vi "S4GUI.vi"(7 "Tab ObsEng":enum32{"Obs", "CCD modes", "Guider", "Eng"}(tab)) -> ()   [LabVIEW 2018] (continued)
            n1734 = call-dynamic "Read State Machine.vi"("error in (no error)"=w3186, "Device in"=w3187) -> ("error out"=w3286:errorcluster, "State Machine.lvclass"=w3288:refnum<class "State Machine.lvclass">, "Device out"=w3289:refnum<class "Channel.lvclass">)  [unwired: 7 in]
            n1735 = call-dynamic "Write State.vi"("error in (no error)"=w3286, "State"=60, "State Machine in"=w3288) -> ("error out"=w3285:errorcluster, "State Machine out"=w3287:refnum<class "State Machine.lvclass">)  [unwired: 7 in]
            n1736 = call-dynamic "Write State Machine.vi"("error in (no error)"=w3285, "State Machine.lvclass"=w3287, "Device in"=w3289) -> ("error out"=w3282:errorcluster, "Device out"=w3283:refnum<class "Channel.lvclass">)  [unwired: 7 in]
            n1737 = call-dynamic "Write Channel.vi"("error in (no error)"=w3282, "Channel.lvclass"=w3283, "Acquisition in"=w3291) -> ("error out"=w3281:errorcluster, "Acquisition out"=w3280:refnum<class "Acquisition.lvclass">)  [unwired: 7 in]
            n1738 = call-dynamic "Write AcquisitionA.vi"("error in (no error)"=w3281, "Acquisition.lvclass"=w3280, "S4ACS_GUI in"=w3293) -> ("error out"=w3217:errorcluster, "S4ACS_GUI out"=w3216:refnum<class "S4GUI.lvclass">)  [unwired: 7 in]
            n1739 = call "Read AcquisitionB.vi"("error in (no error)"=w3217, "S4ACS_GUI in"=w3216) -> ("error out"=w3259:errorcluster, "Acquisition.lvclass"=w3257:refnum<class "Acquisition.lvclass">, "S4ACS_GUI out"=w3256:refnum<class "S4GUI.lvclass">)  [unwired: 7 in]
            n1740 = call-dynamic "Read Channel.vi"("error in (no error)"=w3259, "Acquisition in"=w3257) -> ("error out"=w3272:errorcluster, "Channel.lvclass"=w3270:refnum<class "Channel.lvclass">, "Acquisition out"=w3258:refnum<class "Acquisition.lvclass">)  [unwired: 7 in]
            n1741 = call "Write section_name.vi"("error in (no error)"=w3272, "section_name"="CCD_ACS2", "Channel in"=w3270) -> ("error out"=w3273:errorcluster, "Channel out"=w3271:refnum<class "Channel.lvclass">)  [unwired: 7 in]
            n1742 = call-dynamic "load config.vi"("error in (no error)"=w3273, "cfg file name"=w3206, "Channel in"=w3271) -> ("error out"=w3201:errorcluster, "Channel out"=w3199:refnum<class "Channel.lvclass">)  [unwired: 7 in]
            n1743 = call-dynamic "save config.vi"("error in (no error)"=w3201, "file config"="lastsaved.cfg", "Channel in"=w3199) -> ("error out"=w3200:errorcluster, "Channel out"=w3198:refnum<class "Channel.lvclass">)  [unwired: 7 in]
            n1744 = call-dynamic "Read State Machine.vi"("error in (no error)"=w3200, "Device in"=w3198) -> ("error out"=w3263:errorcluster, "State Machine.lvclass"=w3261:refnum<class "State Machine.lvclass">, "Device out"=w3260:refnum<class "Channel.lvclass">)  [unwired: 7 in]
            n1745 = call-dynamic "Write State.vi"("error in (no error)"=w3263, "State"=60, "State Machine in"=w3261) -> ("error out"=w3264:errorcluster, "State Machine out"=w3262:refnum<class "State Machine.lvclass">)  [unwired: 7 in]
            n1746 = call-dynamic "Write State Machine.vi"("error in (no error)"=w3264, "State Machine.lvclass"=w3262, "Device in"=w3260) -> ("error out"=w3267:errorcluster, "Device out"=w3266:refnum<class "Channel.lvclass">)  [unwired: 7 in]
            n1747 = call-dynamic "Write Channel.vi"("error in (no error)"=w3267, "Channel.lvclass"=w3266, "Acquisition in"=w3258) -> ("error out"=w3268:errorcluster, "Acquisition out"=w3269:refnum<class "Acquisition.lvclass">)  [unwired: 7 in]
            n1748 = call "Write AcquisitionB.vi"("error in (no error)"=w3268, "Acquisition.lvclass"=w3269, "S4ACS_GUI in"=w3256) -> ("error out"=w3215:errorcluster, "S4ACS_GUI out"=w3214:refnum<class "S4GUI.lvclass">)  [unwired: 7 in]
            n1749 = call-dynamic "Read AcquisitionC.vi"("error in (no error)"=w3215, "S4ACS_GUI in"=w3214) -> ("error out"=w3252:errorcluster, "Acquisition.lvclass"=w3254:refnum<class "Acquisition.lvclass">, "S4ACS_GUI out"=w3255:refnum<class "S4GUI.lvclass">)  [unwired: 7 in]
            n1750 = call-dynamic "Read Channel.vi"("error in (no error)"=w3252, "Acquisition in"=w3254) -> ("error out"=w3239:errorcluster, "Channel.lvclass"=w3241:refnum<class "Channel.lvclass">, "Acquisition out"=w3253:refnum<class "Acquisition.lvclass">)  [unwired: 7 in]
            n1751 = call "Write section_name.vi"("error in (no error)"=w3239, "section_name"="CCD_ACS3", "Channel in"=w3241) -> ("error out"=w3238:errorcluster, "Channel out"=w3240:refnum<class "Channel.lvclass">)  [unwired: 7 in]
            n1752 = call-dynamic "load config.vi"("error in (no error)"=w3238, "cfg file name"=w3206, "Channel in"=w3240) -> ("error out"=w3196:errorcluster, "Channel out"=w3194:refnum<class "Channel.lvclass">)  [unwired: 7 in]
            n1753 = call-dynamic "save config.vi"("error in (no error)"=w3196, "file config"="lastsaved.cfg", "Channel in"=w3194) -> ("error out"=w3195:errorcluster, "Channel out"=w3193:refnum<class "Channel.lvclass">)  [unwired: 7 in]
            n1754 = call-dynamic "Read State Machine.vi"("error in (no error)"=w3195, "Device in"=w3193) -> ("error out"=w3248:errorcluster, "State Machine.lvclass"=w3250:refnum<class "State Machine.lvclass">, "Device out"=w3251:refnum<class "Channel.lvclass">)  [unwired: 7 in]
            n1755 = call-dynamic "Write State.vi"("error in (no error)"=w3248, "State"=60, "State Machine in"=w3250) -> ("error out"=w3247:errorcluster, "State Machine out"=w3249:refnum<class "State Machine.lvclass">)  [unwired: 7 in]
            n1756 = call-dynamic "Write State Machine.vi"("error in (no error)"=w3247, "State Machine.lvclass"=w3249, "Device in"=w3251) -> ("error out"=w3244:errorcluster, "Device out"=w3245:refnum<class "Channel.lvclass">)  [unwired: 7 in]
            n1757 = call-dynamic "Write Channel.vi"("error in (no error)"=w3244, "Channel.lvclass"=w3245, "Acquisition in"=w3253) -> ("error out"=w3243:errorcluster, "Acquisition out"=w3242:refnum<class "Acquisition.lvclass">)  [unwired: 7 in]
            n1758 = call-dynamic "Write AcquisitionC.vi"("error in (no error)"=w3243, "Acquisition.lvclass"=w3242, "S4ACS_GUI in"=w3255) -> ("error out"=w3213:errorcluster, "S4ACS_GUI out"=w3212:refnum<class "S4GUI.lvclass">)  [unwired: 7 in]
            n1759 = call-dynamic "Read AcquisitionD.vi"("error in (no error)"=w3213, "S4ACS_GUI in"=w3212) -> ("error out"=w3221:errorcluster, "Acquisition.lvclass"=w3219:refnum<class "Acquisition.lvclass">, "S4ACS_GUI out"=w3218:refnum<class "S4GUI.lvclass">)  [unwired: 7 in]
            n1760 = call-dynamic "Read Channel.vi"("error in (no error)"=w3221, "Acquisition in"=w3219) -> ("error out"=w3234:errorcluster, "Channel.lvclass"=w3232:refnum<class "Channel.lvclass">, "Acquisition out"=w3220:refnum<class "Acquisition.lvclass">)  [unwired: 7 in]
            n1761 = call "Write section_name.vi"("error in (no error)"=w3234, "section_name"="CCD_ACS4", "Channel in"=w3232) -> ("error out"=w3235:errorcluster, "Channel out"=w3233:refnum<class "Channel.lvclass">)  [unwired: 7 in]
            n1762 = call-dynamic "load config.vi"("error in (no error)"=w3235, "cfg file name"=w3206, "Channel in"=w3233) -> ("error out"=w3192:errorcluster, "Channel out"=w3190:refnum<class "Channel.lvclass">)  [unwired: 7 in]
            n1763 = call-dynamic "save config.vi"("error in (no error)"=w3192, "file config"="lastsaved.cfg", "Channel in"=w3190) -> ("error out"=w3191:errorcluster, "Channel out"=w3189:refnum<class "Channel.lvclass">)  [unwired: 7 in]
            n1764 = call-dynamic "Read State Machine.vi"("error in (no error)"=w3191, "Device in"=w3189) -> ("error out"=w3225:errorcluster, "State Machine.lvclass"=w3223:refnum<class "State Machine.lvclass">, "Device out"=w3222:refnum<class "Channel.lvclass">)  [unwired: 7 in]
            n1765 = call-dynamic "Write State.vi"("error in (no error)"=w3225, "State"=60, "State Machine in"=w3223) -> ("error out"=w3226:errorcluster, "State Machine out"=w3224:refnum<class "State Machine.lvclass">)  [unwired: 7 in]
            n1766 = call-dynamic "Write State Machine.vi"("error in (no error)"=w3226, "State Machine.lvclass"=w3224, "Device in"=w3222) -> ("error out"=w3229:errorcluster, "Device out"=w3228:refnum<class "Channel.lvclass">)  [unwired: 7 in]
            n1767 = call-dynamic "Write Channel.vi"("error in (no error)"=w3229, "Channel.lvclass"=w3228, "Acquisition in"=w3220) -> ("error out"=w3230:errorcluster, "Acquisition out"=w3231:refnum<class "Acquisition.lvclass">)  [unwired: 7 in]
            n1768 = call-dynamic "Write AcquisitionD.vi"("error in (no error)"=w3230, "Acquisition.lvclass"=w3231, "S4ACS_GUI in"=w3218) -> ("error out"=w3209:errorcluster, "S4ACS_GUI out"=w3211:refnum<class "S4GUI.lvclass">)  [unwired: 7 in]
            n1769 = Unbundle By Name(w3162) -> ("INITIAL_LINE"=w3183:u16, "INITIAL_COLUMN"=w3182:u16, "FINAL_LINE"=w3181:u16, "FINAL_COLUMN"=w3180:u16, "VBIN"=w3179:u16, "HBIN"=w3178:u16, "PREAMP"=w3177:u8, "EM_GAIN"=w3176:u16, "READOUT_RATE"=w3175:u8, "SHUTTER_OPENING_TIME"=w3174:u16, "SHUTTER_CLOSING_TIME"=w3173:u16, "VERTICAL_SHIFT_SPEED"=w3163:u8, "READ_MODE"=w3172:u8, "VERTICAL_CLOCK_VOLTAGE"=w3171:u8, "AD_CHANNEL"=w3170:u32, "SHUTTER_MODE"=w3169:u8, "SHUTTER_TTL"=w3168:u8, "TRIGGER_MODE"=w3167:u8, "FRAME_TRANSFER"=w3166:bool, "ACQUISITION_MODE"=w3165:u8, "EM_MODE"=w3164:u8)
            n1770 = call "Write cfg file.vi"("error in (no error)"=w3209, "cfg file"=w3206, "S4ACS_GUI in"=w3211) -> ("error out"=w3208:errorcluster, "S4ACS_GUI out"=w3210:refnum<class "S4GUI.lvclass">)  [unwired: 7 in]
            n1771 = local read "Input Cluster"() -> (w3185:T8)
            n1772 = Bundle By Name(cluster=w3185, "Parameters.Image \nInitial Line"=w3183, "Parameters.Image\nInitial Column"=w3182, "Parameters.Image\nFinal Line"=w3181, "Parameters.Image\nFInal Column"=w3180, "Parameters.Vertical\nBinning"=w3179, "Parameters.Horizontal\nBinning"=w3178, "Parameters.Pre-amplification\nGain"=w3177, "Parameters.CCD\nEM Gain"=w3176, "Parameters.Readout\nRate"=w3175, "Parameters.Shutter\nOpenning Time"=w3174, "Parameters.Shutter\nClosing Time"=w3173, "Parameters.Vertical\nShift Speed"=w3163, "Parameters.Read\nMode"=w3172, "Parameters.Vertical\nClock Voltage"=w3171, "Parameters.A/D \nChannel"=w3170, "Parameters.Shutter\nMode"=w3169, "Parameters.Shutter\nTTL"=w3168, "Parameters.Trigger\nMode"=w3167, "Parameters.Frame\nTransfer"=w3166, "Parameters.Acquisition\nMode"=w3165, "Parameters.CCD \nEM Mode"=w3164) -> (w3184:T8)
            n1773 = local write "Input Cluster"(w3184) -> ()
          }
          frame True {
          }
        }
      }
      event "Save As Button": Value Change {
        n1774 = event-data() -> ()  [unwired: 1 in, 6 out]
        n1775 = disable-structure shown="Enabled" {
          disable-tunnel: [w3310 w3322] -> w3299
          disable-tunnel: w3298 -> [w3309 _]
          disable-tunnel: [w3303 w3320] -> w3297
          frame Disabled {
            n1776 = String To Path(string="C:\\Users\\observer\\sparc4\\s4gui\\Config" ("default name")) -> (path=w3305:path)
            n1777 = call "File Dialog2"("start path"=w3305, "prompt"="Select file...", "button label"="Save", "default name"="lastsaved.cfg", "error in"=w3309, "pattern (all files)"="*.cfg") -> ("selected path"=w3304:path, "cancelled"=w3310:bool, "error out"=→"error out 3":errorcluster)  [unwired: 6 in, 1 out]
            n1778 = Strip Path(path=w3304) -> (name=w3303:string)  [unwired: 1 out]
          }
          frame Enabled {
            w3324 = ".cfg" ("regular expression")
            n1779 = Match Pattern(string="savefile", regular expression=w3324) -> (before substring=w3319:string, match substring=w3323:string)  [unwired: 1 in, 2 out]
            n1780 = String Length(string=w3319) -> (length=w3318:i32)
            n1781 = Equal?(x=w3323, y=w3324) -> (x = y?=w3314:bool)
            n1782 = Less?(x=w3318, y=20) -> (x < y?=w3315:bool)
            n1783 = And(x=w3315, y=w3314) -> (x .and. y?=w3316:bool)
            n1784 = case shown="False" w3316 {
              tunnel: w3319 -> [_ w3337]
              tunnel: w3323 -> [_ w3336]
              tunnel: [TRUE ("cancelled") FALSE ("cancelled")] -> w3322
              tunnel: [w3327 w3335] -> w3320
              tunnel: [w3327 w3335] -> w3321
              frame False {
                w3327 = "lastsaved.cfg" ("savefile")
                n1785 = One Button Dialog(message="Invalid file name!\nFile name length must be less than 20 characters\nand must contain .cfg ending." ("savefile")) -> ()  [unwired: 1 in, 1 out]
              }
              frame True {
                n1786 = call <vilib>:"Trim Whitespace.vi"("string"=w3337) -> ("trimmed string"=w3334:string)  [unwired: 1 in]
                n1787 = call <vilib>:"Space Constant.vi"() -> ("String"=w3332:string)
                n1788 = To Lower Case(string=w3334) -> (all lower case string=w3330:string)
                n1789 = Search and Replace String(replace all?=TRUE ("replace all? (F)"), input string=w3330, search string=w3332, replace string="" ("replace string (\"\")")) -> (result string=w3329:string)  [unwired: 4 in, 3 out]
                n1790 = Concatenate Strings(w3329, w3336) -> (w3335:string)
              }
            }
            n1791 = local write "savefile"(w3321) -> ()
          }
        }
        n1792 = case shown="False" w3299 {
          tunnel: w3302 -> [w3403 w3405]
          tunnel: [w3351 w3405] -> w3301
          tunnel: [w3349 w3404] -> w3300
          tunnel: w3298 -> [w3348 w3404]
          tunnel: w3297 -> [w3347 _]
          frame False {
            n1793 = call-dynamic "Read AcquisitionA.vi"("error in (no error)"=w3348, "S4ACS_GUI in"=w3403) -> ("error out"=w3399:errorcluster, "Acquisition.lvclass"=w3401:refnum<class "Acquisition.lvclass">, "S4ACS_GUI out"=w3402:refnum<class "S4GUI.lvclass">)  [unwired: 7 in]
            n1794 = call-dynamic "Read Channel.vi"("error in (no error)"=w3399, "Acquisition in"=w3401) -> ("error out"=w3394:errorcluster, "Channel.lvclass"=w3396:refnum<class "Channel.lvclass">, "Acquisition out"=w3400:refnum<class "Acquisition.lvclass">)  [unwired: 7 in]
            n1795 = call "Write section_name.vi"("error in (no error)"=w3394, "section_name"="CCD_ACS1", "Channel in"=w3396) -> ("error out"=w3393:errorcluster, "Channel out"=w3395:refnum<class "Channel.lvclass">)  [unwired: 7 in]
            n1796 = call-dynamic "save config.vi"("error in (no error)"=w3393, "file config"=w3347, "Channel in"=w3395) -> ("error out"=w3345:errorcluster, "Channel out"=w3346:refnum<class "Channel.lvclass">)  [unwired: 7 in]
            n1797 = call-dynamic "Write Channel.vi"("error in (no error)"=w3345, "Channel.lvclass"=w3346, "Acquisition in"=w3400) -> ("error out"=w3398:errorcluster, "Acquisition out"=w3397:refnum<class "Acquisition.lvclass">)  [unwired: 7 in]
            n1798 = call-dynamic "Write AcquisitionA.vi"("error in (no error)"=w3398, "Acquisition.lvclass"=w3397, "S4ACS_GUI in"=w3402) -> ("error out"=w3358:errorcluster, "S4ACS_GUI out"=w3357:refnum<class "S4GUI.lvclass">)  [unwired: 7 in]
            n1799 = call "Read AcquisitionB.vi"("error in (no error)"=w3358, "S4ACS_GUI in"=w3357) -> ("error out"=w3384:errorcluster, "Acquisition.lvclass"=w3382:refnum<class "Acquisition.lvclass">, "S4ACS_GUI out"=w3381:refnum<class "S4GUI.lvclass">)  [unwired: 7 in]
            n1800 = call-dynamic "Read Channel.vi"("error in (no error)"=w3384, "Acquisition in"=w3382) -> ("error out"=w3389:errorcluster, "Channel.lvclass"=w3387:refnum<class "Channel.lvclass">, "Acquisition out"=w3383:refnum<class "Acquisition.lvclass">)  [unwired: 7 in]
            n1801 = call "Write section_name.vi"("error in (no error)"=w3389, "section_name"="CCD_ACS2", "Channel in"=w3387) -> ("error out"=w3390:errorcluster, "Channel out"=w3388:refnum<class "Channel.lvclass">)  [unwired: 7 in]
            n1802 = call-dynamic "save config.vi"("error in (no error)"=w3390, "file config"=w3347, "Channel in"=w3388) -> ("error out"=w3339:errorcluster, "Channel out"=w3340:refnum<class "Channel.lvclass">)  [unwired: 7 in]
            n1803 = call-dynamic "Write Channel.vi"("error in (no error)"=w3339, "Channel.lvclass"=w3340, "Acquisition in"=w3383) -> ("error out"=w3385:errorcluster, "Acquisition out"=w3386:refnum<class "Acquisition.lvclass">)  [unwired: 7 in]
            n1804 = call "Write AcquisitionB.vi"("error in (no error)"=w3385, "Acquisition.lvclass"=w3386, "S4ACS_GUI in"=w3381) -> ("error out"=w3356:errorcluster, "S4ACS_GUI out"=w3355:refnum<class "S4GUI.lvclass">)  [unwired: 7 in]
            n1805 = call-dynamic "Read AcquisitionC.vi"("error in (no error)"=w3356, "S4ACS_GUI in"=w3355) -> ("error out"=w3377:errorcluster, "Acquisition.lvclass"=w3379:refnum<class "Acquisition.lvclass">, "S4ACS_GUI out"=w3380:refnum<class "S4GUI.lvclass">)  [unwired: 7 in]
            n1806 = call-dynamic "Read Channel.vi"("error in (no error)"=w3377, "Acquisition in"=w3379) -> ("error out"=w3372:errorcluster, "Channel.lvclass"=w3374:refnum<class "Channel.lvclass">, "Acquisition out"=w3378:refnum<class "Acquisition.lvclass">)  [unwired: 7 in]
            n1807 = call "Write section_name.vi"("error in (no error)"=w3372, "section_name"="CCD_ACS3", "Channel in"=w3374) -> ("error out"=w3371:errorcluster, "Channel out"=w3373:refnum<class "Channel.lvclass">)  [unwired: 7 in]
            n1808 = call-dynamic "save config.vi"("error in (no error)"=w3371, "file config"=w3347, "Channel in"=w3373) -> ("error out"=w3341:errorcluster, "Channel out"=w3342:refnum<class "Channel.lvclass">)  [unwired: 7 in]
            n1809 = call-dynamic "Write Channel.vi"("error in (no error)"=w3341, "Channel.lvclass"=w3342, "Acquisition in"=w3378) -> ("error out"=w3376:errorcluster, "Acquisition out"=w3375:refnum<class "Acquisition.lvclass">)  [unwired: 7 in]
            n1810 = call-dynamic "Write AcquisitionC.vi"("error in (no error)"=w3376, "Acquisition.lvclass"=w3375, "S4ACS_GUI in"=w3380) -> ("error out"=w3354:errorcluster, "S4ACS_GUI out"=w3353:refnum<class "S4GUI.lvclass">)  [unwired: 7 in]
            n1811 = call-dynamic "Read AcquisitionD.vi"("error in (no error)"=w3354, "S4ACS_GUI in"=w3353) -> ("error out"=w3362:errorcluster, "Acquisition.lvclass"=w3360:refnum<class "Acquisition.lvclass">, "S4ACS_GUI out"=w3359:refnum<class "S4GUI.lvclass">)  [unwired: 7 in]
            n1812 = call-dynamic "Read Channel.vi"("error in (no error)"=w3362, "Acquisition in"=w3360) -> ("error out"=w3367:errorcluster, "Channel.lvclass"=w3365:refnum<class "Channel.lvclass">, "Acquisition out"=w3361:refnum<class "Acquisition.lvclass">)  [unwired: 7 in]
            n1813 = call "Write section_name.vi"("error in (no error)"=w3367, "section_name"="CCD_ACS4", "Channel in"=w3365) -> ("error out"=w3368:errorcluster, "Channel out"=w3366:refnum<class "Channel.lvclass">)  [unwired: 7 in]
            n1814 = call-dynamic "save config.vi"("error in (no error)"=w3368, "file config"=w3347, "Channel in"=w3366) -> ("error out"=w3343:errorcluster, "Channel out"=w3344:refnum<class "Channel.lvclass">)  [unwired: 7 in]
            n1815 = call-dynamic "Write Channel.vi"("error in (no error)"=w3343, "Channel.lvclass"=w3344, "Acquisition in"=w3361) -> ("error out"=w3363:errorcluster, "Acquisition out"=w3364:refnum<class "Acquisition.lvclass">)  [unwired: 7 in]
            n1816 = call-dynamic "Write AcquisitionD.vi"("error in (no error)"=w3363, "Acquisition.lvclass"=w3364, "S4ACS_GUI in"=w3359) -> ("error out"=w3350:errorcluster, "S4ACS_GUI out"=w3352:refnum<class "S4GUI.lvclass">)  [unwired: 7 in]
            n1817 = call "Write cfg file.vi"("error in (no error)"=w3350, "cfg file"=w3347, "S4ACS_GUI in"=w3352) -> ("error out"=w3349:errorcluster, "S4ACS_GUI out"=w3351:refnum<class "S4GUI.lvclass">)  [unwired: 7 in]
          }
          frame True {
          }
        }
      }
      event "Load Default Button": Value Change {
        w3450 = "default.cfg" ("cfg file name")
        n1818 = event-data() -> ()  [unwired: 1 in, 6 out]
        n1819 = call-dynamic "Read AcquisitionA.vi"("error in (no error)"=w3540, "S4ACS_GUI in"=w3541) -> ("error out"=w3536:errorcluster, "Acquisition.lvclass"=w3538:refnum<class "Acquisition.lvclass">, "S4ACS_GUI out"=w3539:refnum<class "S4GUI.lvclass">)  [unwired: 7 in]
        n1820 = call-dynamic "Read Channel.vi"("error in (no error)"=w3536, "Acquisition in"=w3538) -> ("error out"=w3523:errorcluster, "Channel.lvclass"=w3525:refnum<class "Channel.lvclass">, "Acquisition out"=w3537:refnum<class "Acquisition.lvclass">)  [unwired: 7 in]
        n1821 = call "Write section_name.vi"("error in (no error)"=w3523, "section_name"="CCD_ACS1", "Channel in"=w3525) -> ("error out"=w3522:errorcluster, "Channel out"=w3524:refnum<class "Channel.lvclass">)  [unwired: 7 in]
        n1822 = call-dynamic "load config.vi"("error in (no error)"=w3522, "cfg file name"=w3450, "Channel in"=w3524) -> ("error out"=w3448:errorcluster, "Channel out"=w3449:refnum<class "Channel.lvclass">)  [unwired: 7 in]
        n1823 = call-dynamic "save config.vi"("error in (no error)"=w3448, "file config"="lastsaved.cfg", "Channel in"=w3449) -> ("error out"=w3407:errorcluster, "Channel out"=w3408:refnum<class "Channel.lvclass">)  [unwired: 7 in]
        n1824 = call-dynamic "Read target cluster.vi"("error in (no error)"=w3407, "Channel in"=w3408) -> ("target cluster"=w3406:T31)  [unwired: 7 in, 2 out]
        n1825 = call-dynamic "Read State Machine.vi"("error in (no error)"=w3407, "Device in"=w3408) -> ("error out"=w3532:errorcluster, "State Machine.lvclass"=w3534:refnum<class "State Machine.lvclass">, "Device out"=w3535:refnum<class "Channel.lvclass">)  [unwired: 7 in]
        n1826 = call-dynamic "Write State.vi"("error in (no error)"=w3532, "State"=60, "State Machine in"=w3534) -> ("error out"=w3531:errorcluster, "State Machine out"=w3533:refnum<class "State Machine.lvclass">)  [unwired: 7 in]
        n1827 = call-dynamic "Write State Machine.vi"("error in (no error)"=w3531, "State Machine.lvclass"=w3533, "Device in"=w3535) -> ("error out"=w3528:errorcluster, "Device out"=w3529:refnum<class "Channel.lvclass">)  [unwired: 7 in]
        n1828 = call-dynamic "Write Channel.vi"("error in (no error)"=w3528, "Channel.lvclass"=w3529, "Acquisition in"=w3537) -> ("error out"=w3527:errorcluster, "Acquisition out"=w3526:refnum<class "Acquisition.lvclass">)  [unwired: 7 in]
        n1829 = call-dynamic "Write AcquisitionA.vi"("error in (no error)"=w3527, "Acquisition.lvclass"=w3526, "S4ACS_GUI in"=w3539) -> ("error out"=w3460:errorcluster, "S4ACS_GUI out"=w3459:refnum<class "S4GUI.lvclass">)  [unwired: 7 in]
        n1830 = call "Read AcquisitionB.vi"("error in (no error)"=w3460, "S4ACS_GUI in"=w3459) -> ("error out"=w3504:errorcluster, "Acquisition.lvclass"=w3502:refnum<class "Acquisition.lvclass">, "S4ACS_GUI out"=w3501:refnum<class "S4GUI.lvclass">)  [unwired: 7 in]
        n1831 = call-dynamic "Read Channel.vi"("error in (no error)"=w3504, "Acquisition in"=w3502) -> ("error out"=w3518:errorcluster, "Channel.lvclass"=w3516:refnum<class "Channel.lvclass">, "Acquisition out"=w3503:refnum<class "Acquisition.lvclass">)  [unwired: 7 in]
        n1832 = call "Write section_name.vi"("error in (no error)"=w3518, "section_name"="CCD_ACS2", "Channel in"=w3516) -> ("error out"=w3519:errorcluster, "Channel out"=w3517:refnum<class "Channel.lvclass">)  [unwired: 7 in]
        n1833 = call-dynamic "load config.vi"("error in (no error)"=w3519, "cfg file name"="default.cfg", "Channel in"=w3517) -> ("error out"=w3445:errorcluster, "Channel out"=w3443:refnum<class "Channel.lvclass">)  [unwired: 7 in]
        n1834 = call-dynamic "save config.vi"("error in (no error)"=w3445, "file config"="lastsaved.cfg", "Channel in"=w3443) -> ("error out"=w3444:errorcluster, "Channel out"=w3442:refnum<class "Channel.lvclass">)  [unwired: 7 in]
        n1835 = call-dynamic "Read State Machine.vi"("error in (no error)"=w3444, "Device in"=w3442) -> ("error out"=w3508:errorcluster, "State Machine.lvclass"=w3506:refnum<class "State Machine.lvclass">, "Device out"=w3505:refnum<class "Channel.lvclass">)  [unwired: 7 in]
        n1836 = call-dynamic "Write State.vi"("error in (no error)"=w3508, "State"=60, "State Machine in"=w3506) -> ("error out"=w3509:errorcluster, "State Machine out"=w3507:refnum<class "State Machine.lvclass">)  [unwired: 7 in]
        n1837 = call-dynamic "Write State Machine.vi"("error in (no error)"=w3509, "State Machine.lvclass"=w3507, "Device in"=w3505) -> ("error out"=w3512:errorcluster, "Device out"=w3511:refnum<class "Channel.lvclass">)  [unwired: 7 in]
        n1838 = call-dynamic "Write Channel.vi"("error in (no error)"=w3512, "Channel.lvclass"=w3511, "Acquisition in"=w3503) -> ("error out"=w3513:errorcluster, "Acquisition out"=w3514:refnum<class "Acquisition.lvclass">)  [unwired: 7 in]
        n1839 = call "Write AcquisitionB.vi"("error in (no error)"=w3513, "Acquisition.lvclass"=w3514, "S4ACS_GUI in"=w3501) -> ("error out"=w3458:errorcluster, "S4ACS_GUI out"=w3457:refnum<class "S4GUI.lvclass">)  [unwired: 7 in]
        n1840 = call-dynamic "Read AcquisitionC.vi"("error in (no error)"=w3458, "S4ACS_GUI in"=w3457) -> ("error out"=w3497:errorcluster, "Acquisition.lvclass"=w3499:refnum<class "Acquisition.lvclass">, "S4ACS_GUI out"=w3500:refnum<class "S4GUI.lvclass">)  [unwired: 7 in]
        n1841 = call-dynamic "Read Channel.vi"("error in (no error)"=w3497, "Acquisition in"=w3499) -> ("error out"=w3483:errorcluster, "Channel.lvclass"=w3485:refnum<class "Channel.lvclass">, "Acquisition out"=w3498:refnum<class "Acquisition.lvclass">)  [unwired: 7 in]
        n1842 = call "Write section_name.vi"("error in (no error)"=w3483, "section_name"="CCD_ACS3", "Channel in"=w3485) -> ("error out"=w3482:errorcluster, "Channel out"=w3484:refnum<class "Channel.lvclass">)  [unwired: 7 in]
        n1843 = call-dynamic "load config.vi"("error in (no error)"=w3482, "cfg file name"="default.cfg", "Channel in"=w3484) -> ("error out"=w3439:errorcluster, "Channel out"=w3440:refnum<class "Channel.lvclass">)  [unwired: 7 in]
        n1844 = call-dynamic "save config.vi"("error in (no error)"=w3439, "file config"="lastsaved.cfg", "Channel in"=w3440) -> ("error out"=w3437:errorcluster, "Channel out"=w3438:refnum<class "Channel.lvclass">)  [unwired: 7 in]
        n1845 = call-dynamic "Read State Machine.vi"("error in (no error)"=w3437, "Device in"=w3438) -> ("error out"=w3493:errorcluster, "State Machine.lvclass"=w3495:refnum<class "State Machine.lvclass">, "Device out"=w3496:refnum<class "Channel.lvclass">)  [unwired: 7 in]
        n1846 = call-dynamic "Write State.vi"("error in (no error)"=w3493, "State"=60, "State Machine in"=w3495) -> ("error out"=w3492:errorcluster, "State Machine out"=w3494:refnum<class "State Machine.lvclass">)  [unwired: 7 in]
        n1847 = call-dynamic "Write State Machine.vi"("error in (no error)"=w3492, "State Machine.lvclass"=w3494, "Device in"=w3496) -> ("error out"=w3489:errorcluster, "Device out"=w3490:refnum<class "Channel.lvclass">)  [unwired: 7 in]
        n1848 = call-dynamic "Write Channel.vi"("error in (no error)"=w3489, "Channel.lvclass"=w3490, "Acquisition in"=w3498) -> ("error out"=w3488:errorcluster, "Acquisition out"=w3487:refnum<class "Acquisition.lvclass">)  [unwired: 7 in]
        n1849 = call-dynamic "Write AcquisitionC.vi"("error in (no error)"=w3488, "Acquisition.lvclass"=w3487, "S4ACS_GUI in"=w3500) -> ("error out"=w3456:errorcluster, "S4ACS_GUI out"=w3455:refnum<class "S4GUI.lvclass">)  [unwired: 7 in]
        n1850 = call-dynamic "Read AcquisitionD.vi"("error in (no error)"=w3456, "S4ACS_GUI in"=w3455) -> ("error out"=w3464:errorcluster, "Acquisition.lvclass"=w3462:refnum<class "Acquisition.lvclass">, "S4ACS_GUI out"=w3461:refnum<class "S4GUI.lvclass">)  [unwired: 7 in]
        n1851 = call-dynamic "Read Channel.vi"("error in (no error)"=w3464, "Acquisition in"=w3462) -> ("error out"=w3478:errorcluster, "Channel.lvclass"=w3476:refnum<class "Channel.lvclass">, "Acquisition out"=w3463:refnum<class "Acquisition.lvclass">)  [unwired: 7 in]
        n1852 = call "Write section_name.vi"("error in (no error)"=w3478, "section_name"="CCD_ACS4", "Channel in"=w3476) -> ("error out"=w3479:errorcluster, "Channel out"=w3477:refnum<class "Channel.lvclass">)  [unwired: 7 in]
        n1853 = call-dynamic "load config.vi"("error in (no error)"=w3479, "cfg file name"="default.cfg", "Channel in"=w3477) -> ("error out"=w3435:errorcluster, "Channel out"=w3434:refnum<class "Channel.lvclass">)  [unwired: 7 in]
        n1854 = call-dynamic "save config.vi"("error in (no error)"=w3435, "file config"="lastsaved.cfg", "Channel in"=w3434) -> ("error out"=w3432:errorcluster, "Channel out"=w3433:refnum<class "Channel.lvclass">)  [unwired: 7 in]
        n1855 = call-dynamic "Read State Machine.vi"("error in (no error)"=w3432, "Device in"=w3433) -> ("error out"=w3468:errorcluster, "State Machine.lvclass"=w3466:refnum<class "State Machine.lvclass">, "Device out"=w3465:refnum<class "Channel.lvclass">)  [unwired: 7 in]
        n1856 = call-dynamic "Write State.vi"("error in (no error)"=w3468, "State"=60, "State Machine in"=w3466) -> ("error out"=w3469:errorcluster, "State Machine out"=w3467:refnum<class "State Machine.lvclass">)  [unwired: 7 in]
        n1857 = call-dynamic "Write State Machine.vi"("error in (no error)"=w3469, "State Machine.lvclass"=w3467, "Device in"=w3465) -> ("error out"=w3472:errorcluster, "Device out"=w3471:refnum<class "Channel.lvclass">)  [unwired: 7 in]
        n1858 = call-dynamic "Write Channel.vi"("error in (no error)"=w3472, "Channel.lvclass"=w3471, "Acquisition in"=w3463) -> ("error out"=w3473:errorcluster, "Acquisition out"=w3474:refnum<class "Acquisition.lvclass">)  [unwired: 7 in]
        n1859 = call-dynamic "Write AcquisitionD.vi"("error in (no error)"=w3473, "Acquisition.lvclass"=w3474, "S4ACS_GUI in"=w3461) -> ("error out"=w3452:errorcluster, "S4ACS_GUI out"=w3454:refnum<class "S4GUI.lvclass">)  [unwired: 7 in]
        n1860 = Unbundle By Name(w3406) -> ("INITIAL_LINE"=w3411:u16, "INITIAL_COLUMN"=w3412:u16, "FINAL_LINE"=w3413:u16, "FINAL_COLUMN"=w3414:u16, "VBIN"=w3415:u16, "HBIN"=w3416:u16, "PREAMP"=w3417:u8, "EM_GAIN"=w3418:u16, "READOUT_RATE"=w3419:u8, "SHUTTER_OPENING_TIME"=w3420:u16, "SHUTTER_CLOSING_TIME"=w3421:u16, "VERTICAL_SHIFT_SPEED"=w3431:u8, "READ_MODE"=w3422:u8, "VERTICAL_CLOCK_VOLTAGE"=w3423:u8, "AD_CHANNEL"=w3424:u32, "SHUTTER_MODE"=w3425:u8, "SHUTTER_TTL"=w3426:u8, "TRIGGER_MODE"=w3427:u8, "FRAME_TRANSFER"=w3428:bool, "ACQUISITION_MODE"=w3429:u8, "EM_MODE"=w3430:u8)
        n1861 = call "Write cfg file.vi"("error in (no error)"=w3452, "cfg file"=w3450, "S4ACS_GUI in"=w3454) -> ("error out"=w3451:errorcluster, "S4ACS_GUI out"=w3453:refnum<class "S4GUI.lvclass">)  [unwired: 7 in]
        n1862 = local read "Input Cluster"() -> (w3409:T8)
        n1863 = Bundle By Name(cluster=w3409, "Parameters.Image \nInitial Line"=w3411, "Parameters.Image\nInitial Column"=w3412, "Parameters.Image\nFinal Line"=w3413, "Parameters.Image\nFInal Column"=w3414, "Parameters.Vertical\nBinning"=w3415, "Parameters.Horizontal\nBinning"=w3416, "Parameters.Pre-amplification\nGain"=w3417, "Parameters.CCD\nEM Gain"=w3418, "Parameters.Readout\nRate"=w3419, "Parameters.Shutter\nOpenning Time"=w3420, "Parameters.Shutter\nClosing Time"=w3421, "Parameters.Vertical\nShift Speed"=w3431, "Parameters.Read\nMode"=w3422, "Parameters.Vertical\nClock Voltage"=w3423, "Parameters.A/D \nChannel"=w3424, "Parameters.Shutter\nMode"=w3425, "Parameters.Shutter\nTTL"=w3426, "Parameters.Trigger\nMode"=w3427, "Parameters.Frame\nTransfer"=w3428, "Parameters.Acquisition\nMode"=w3429, "Parameters.CCD \nEM Mode"=w3430) -> (w3410:T8)
        n1864 = local write "Input Cluster"(w3410) -> ()
      }
      event "Restore Default ch2": Value Change {
        n1865 = event-data() -> ()  [unwired: 1 in, 6 out]
        n1866 = call "Read AcquisitionB.vi"("error in (no error)"=w3572, "S4ACS_GUI in"=w3573) -> ("error out"=w3568:errorcluster, "Acquisition.lvclass"=w3570:refnum<class "Acquisition.lvclass">, "S4ACS_GUI out"=w3571:refnum<class "S4GUI.lvclass">)  [unwired: 7 in]
        n1867 = call-dynamic "Read Channel.vi"("error in (no error)"=w3568, "Acquisition in"=w3570) -> ("error out"=w3555:errorcluster, "Channel.lvclass"=w3557:refnum<class "Channel.lvclass">, "Acquisition out"=w3569:refnum<class "Acquisition.lvclass">)  [unwired: 7 in]
        n1868 = call "Write section_name.vi"("error in (no error)"=w3555, "section_name"="CCD_ACS2", "Channel in"=w3557) -> ("error out"=w3554:errorcluster, "Channel out"=w3556:refnum<class "Channel.lvclass">)  [unwired: 7 in]
        n1869 = call-dynamic "load config.vi"("error in (no error)"=w3554, "cfg file name"="default.cfg", "Channel in"=w3556) -> ("error out"=w3552:errorcluster, "Channel out"=w3553:refnum<class "Channel.lvclass">)  [unwired: 7 in]
        n1870 = call-dynamic "Read State Machine.vi"("error in (no error)"=w3552, "Device in"=w3553) -> ("error out"=w3564:errorcluster, "State Machine.lvclass"=w3566:refnum<class "State Machine.lvclass">, "Device out"=w3567:refnum<class "Channel.lvclass">)  [unwired: 7 in]
        n1871 = call-dynamic "Write State.vi"("error in (no error)"=w3564, "State"=60, "State Machine in"=w3566) -> ("error out"=w3563:errorcluster, "State Machine out"=w3565:refnum<class "State Machine.lvclass">)  [unwired: 7 in]
        n1872 = call-dynamic "Write State Machine.vi"("error in (no error)"=w3563, "State Machine.lvclass"=w3565, "Device in"=w3567) -> ("error out"=w3548:errorcluster, "Device out"=w3545:refnum<class "Channel.lvclass">)  [unwired: 7 in]
        n1873 = call "Write section_name.vi"("error in (no error)"=w3548, "section_name"="CCD_ACS2", "Channel in"=w3545) -> ("error out"=w3549:errorcluster, "Channel out"=w3544:refnum<class "Channel.lvclass">)  [unwired: 7 in]
        n1874 = call-dynamic "save config.vi"("error in (no error)"=w3549, "file config"="lastsaved.cfg", "Channel in"=w3544) -> ("error out"=w3547:errorcluster, "Channel out"=w3543:refnum<class "Channel.lvclass">)  [unwired: 7 in]
        n1875 = call-dynamic "Write Channel.vi"("error in (no error)"=w3547, "Channel.lvclass"=w3543, "Acquisition in"=w3569) -> ("error out"=w3561:errorcluster, "Acquisition out"=w3560:refnum<class "Acquisition.lvclass">)  [unwired: 7 in]
        n1876 = call "Write AcquisitionB.vi"("error in (no error)"=w3561, "Acquisition.lvclass"=w3560, "S4ACS_GUI in"=w3571) -> ("error out"=w3559:errorcluster, "S4ACS_GUI out"=w3550:refnum<class "S4GUI.lvclass">)  [unwired: 7 in]
      }
      event "Restore Default ch3": Value Change {
        n1877 = event-data() -> ()  [unwired: 1 in, 6 out]
        n1878 = call-dynamic "Read AcquisitionC.vi"("error in (no error)"=w3604, "S4ACS_GUI in"=w3605) -> ("error out"=w3600:errorcluster, "Acquisition.lvclass"=w3602:refnum<class "Acquisition.lvclass">, "S4ACS_GUI out"=w3603:refnum<class "S4GUI.lvclass">)  [unwired: 7 in]
        n1879 = call-dynamic "Read Channel.vi"("error in (no error)"=w3600, "Acquisition in"=w3602) -> ("error out"=w3587:errorcluster, "Channel.lvclass"=w3589:refnum<class "Channel.lvclass">, "Acquisition out"=w3601:refnum<class "Acquisition.lvclass">)  [unwired: 7 in]
        n1880 = call "Write section_name.vi"("error in (no error)"=w3587, "section_name"="CCD_ACS3", "Channel in"=w3589) -> ("error out"=w3586:errorcluster, "Channel out"=w3588:refnum<class "Channel.lvclass">)  [unwired: 7 in]
        n1881 = call-dynamic "load config.vi"("error in (no error)"=w3586, "cfg file name"="default.cfg", "Channel in"=w3588) -> ("error out"=w3584:errorcluster, "Channel out"=w3585:refnum<class "Channel.lvclass">)  [unwired: 7 in]
        n1882 = call-dynamic "Read State Machine.vi"("error in (no error)"=w3584, "Device in"=w3585) -> ("error out"=w3596:errorcluster, "State Machine.lvclass"=w3598:refnum<class "State Machine.lvclass">, "Device out"=w3599:refnum<class "Channel.lvclass">)  [unwired: 7 in]
        n1883 = call-dynamic "Write State.vi"("error in (no error)"=w3596, "State"=60, "State Machine in"=w3598) -> ("error out"=w3595:errorcluster, "State Machine out"=w3597:refnum<class "State Machine.lvclass">)  [unwired: 7 in]
        n1884 = call-dynamic "Write State Machine.vi"("error in (no error)"=w3595, "State Machine.lvclass"=w3597, "Device in"=w3599) -> ("error out"=w3575:errorcluster, "Device out"=w3577:refnum<class "Channel.lvclass">)  [unwired: 7 in]
        n1885 = call "Write section_name.vi"("error in (no error)"=w3575, "section_name"="CCD_ACS3", "Channel in"=w3577) -> ("error out"=w3581:errorcluster, "Channel out"=w3576:refnum<class "Channel.lvclass">)  [unwired: 7 in]
        n1886 = call-dynamic "save config.vi"("error in (no error)"=w3581, "file config"="lastsaved.cfg", "Channel in"=w3576) -> ("error out"=w3574:errorcluster, "Channel out"=w3578:refnum<class "Channel.lvclass">)  [unwired: 7 in]
        n1887 = call-dynamic "Write Channel.vi"("error in (no error)"=w3574, "Channel.lvclass"=w3578, "Acquisition in"=w3601) -> ("error out"=w3593:errorcluster, "Acquisition out"=w3592:refnum<class "Acquisition.lvclass">)  [unwired: 7 in]
        n1888 = call-dynamic "Write AcquisitionC.vi"("error in (no error)"=w3593, "Acquisition.lvclass"=w3592, "S4ACS_GUI in"=w3603) -> ("error out"=w3591:errorcluster, "S4ACS_GUI out"=w3582:refnum<class "S4GUI.lvclass">)  [unwired: 7 in]
      }
      event "Restore Default ch4": Value Change {
        n1889 = event-data() -> ()  [unwired: 1 in, 6 out]
        n1890 = call-dynamic "Read AcquisitionD.vi"("error in (no error)"=w3636, "S4ACS_GUI in"=w3637) -> ("error out"=w3632:errorcluster, "Acquisition.lvclass"=w3634:refnum<class "Acquisition.lvclass">, "S4ACS_GUI out"=w3635:refnum<class "S4GUI.lvclass">)  [unwired: 7 in]
        n1891 = call-dynamic "Read Channel.vi"("error in (no error)"=w3632, "Acquisition in"=w3634) -> ("error out"=w3619:errorcluster, "Channel.lvclass"=w3621:refnum<class "Channel.lvclass">, "Acquisition out"=w3633:refnum<class "Acquisition.lvclass">)  [unwired: 7 in]
        n1892 = call "Write section_name.vi"("error in (no error)"=w3619, "section_name"="CCD_ACS4", "Channel in"=w3621) -> ("error out"=w3618:errorcluster, "Channel out"=w3620:refnum<class "Channel.lvclass">)  [unwired: 7 in]
        n1893 = call-dynamic "load config.vi"("error in (no error)"=w3618, "cfg file name"="default.cfg", "Channel in"=w3620) -> ("error out"=w3616:errorcluster, "Channel out"=w3617:refnum<class "Channel.lvclass">)  [unwired: 7 in]
        n1894 = call-dynamic "Read State Machine.vi"("error in (no error)"=w3616, "Device in"=w3617) -> ("error out"=w3628:errorcluster, "State Machine.lvclass"=w3630:refnum<class "State Machine.lvclass">, "Device out"=w3631:refnum<class "Channel.lvclass">)  [unwired: 7 in]
        n1895 = call-dynamic "Write State.vi"("error in (no error)"=w3628, "State"=60, "State Machine in"=w3630) -> ("error out"=w3627:errorcluster, "State Machine out"=w3629:refnum<class "State Machine.lvclass">)  [unwired: 7 in]
        n1896 = call-dynamic "Write State Machine.vi"("error in (no error)"=w3627, "State Machine.lvclass"=w3629, "Device in"=w3631) -> ("error out"=w3607:errorcluster, "Device out"=w3610:refnum<class "Channel.lvclass">)  [unwired: 7 in]
        n1897 = call "Write section_name.vi"("error in (no error)"=w3607, "section_name"="CCD_ACS4", "Channel in"=w3610) -> ("error out"=w3613:errorcluster, "Channel out"=w3609:refnum<class "Channel.lvclass">)  [unwired: 7 in]
        n1898 = call-dynamic "save config.vi"("error in (no error)"=w3613, "file config"="lastsaved.cfg", "Channel in"=w3609) -> ("error out"=w3606:errorcluster, "Channel out"=w3608:refnum<class "Channel.lvclass">)  [unwired: 7 in]
        n1899 = call-dynamic "Write Channel.vi"("error in (no error)"=w3606, "Channel.lvclass"=w3608, "Acquisition in"=w3633) -> ("error out"=w3625:errorcluster, "Acquisition out"=w3624:refnum<class "Acquisition.lvclass">)  [unwired: 7 in]
        n1900 = call-dynamic "Write AcquisitionD.vi"("error in (no error)"=w3625, "Acquisition.lvclass"=w3624, "S4ACS_GUI in"=w3635) -> ("error out"=w3623:errorcluster, "S4ACS_GUI out"=w3614:refnum<class "S4GUI.lvclass">)  [unwired: 7 in]
      }
      event "Copy to Input ch1": Value Change {
        w3638 = T12."Enabled" ("Disabled")
        n1901 = event-data() -> ()  [unwired: 1 in, 6 out]
        n1902 = call-dynamic "Read AcquisitionA.vi"("error in (no error)"=w3671, "S4ACS_GUI in"=w3672) -> ("error out"=w3667:errorcluster, "Acquisition.lvclass"=w3670:refnum<class "Acquisition.lvclass">, "S4ACS_GUI out"=w3639:refnum<class "S4GUI.lvclass">)  [unwired: 7 in]
        n1903 = call-dynamic "Read Channel.vi"("error in (no error)"=w3667, "Acquisition in"=w3670) -> ("error out"=w3666:errorcluster, "Channel.lvclass"=w3669:refnum<class "Channel.lvclass">)  [unwired: 7 in, 1 out]
        n1904 = call-dynamic "Read Interface.vi"("error in (no error)"=w3666, "Channel in"=w3669) -> ("error out"=w3665:errorcluster, "Interface.lvclass"=w3668:refnum<class "Interface.lvclass">)  [unwired: 7 in, 1 out]
        n1905 = call-dynamic "Get CCD_Config.vi"("error in (no error)"=w3665, "Interface in"=w3668) -> ("error out"=w3662:errorcluster, "output cluster"=w3661:T31)  [unwired: 7 in, 1 out]
        n1906 = Unbundle By Name(w3661) -> ("INITIAL_LINE"=w3660:u16, "INITIAL_COLUMN"=w3659:u16, "FINAL_LINE"=w3658:u16, "FINAL_COLUMN"=w3657:u16, "VBIN"=w3656:u16, "HBIN"=w3655:u16, "PREAMP"=w3654:u8, "EM_GAIN"=w3653:u16, "READOUT_RATE"=w3652:u8, "SHUTTER_OPENING_TIME"=w3651:u16, "SHUTTER_CLOSING_TIME"=w3650:u16, "VERTICAL_SHIFT_SPEED"=w3649:u8, "READ_MODE"=w3648:u8, "VERTICAL_CLOCK_VOLTAGE"=w3647:u8, "AD_CHANNEL"=w3646:u32, "SHUTTER_MODE"=w3645:u8, "SHUTTER_TTL"=w3644:u8, "TRIGGER_MODE"=w3643:u8, "FRAME_TRANSFER"=w3642:bool, "ACQUISITION_MODE"=w3641:u8, "EM_MODE"=w3640:u8)
        n1907 = local read "Input Cluster"() -> (w3664:T8)
        n1908 = Bundle By Name(cluster=w3664, "Parameters.Image \nInitial Line"=w3660, "Parameters.Image\nInitial Column"=w3659, "Parameters.Image\nFinal Line"=w3658, "Parameters.Image\nFInal Column"=w3657, "Parameters.Vertical\nBinning"=w3656, "Parameters.Horizontal\nBinning"=w3655, "Parameters.Pre-amplification\nGain"=w3654, "Parameters.CCD\nEM Gain"=w3653, "Parameters.Readout\nRate"=w3652, "Parameters.Shutter\nOpenning Time"=w3651, "Parameters.Shutter\nClosing Time"=w3650, "Parameters.Vertical\nShift Speed"=w3649, "Parameters.Read\nMode"=w3648, "Parameters.Vertical\nClock Voltage"=w3647, "Parameters.A/D \nChannel"=w3646, "Parameters.Shutter\nMode"=w3645, "Parameters.Shutter\nTTL"=w3644, "Parameters.Trigger\nMode"=w3643, "Parameters.Frame\nTransfer"=w3642, "Parameters.Acquisition\nMode"=w3641, "Parameters.CCD \nEM Mode"=w3640) -> (w3663:T8)
        n1909 = local write "Input Cluster"(w3663) -> ()
        n1910 = property on="Set from Input ch1" class="Bool"("DisabledEnum"=w3638) -> ()  [unwired: 2 in, 2 out]
        n1911 = property on="Set from Input ch3" class="Bool"("DisabledEnum"=w3638) -> ()  [unwired: 2 in, 2 out]
        n1912 = property on="Set from Input ch2" class="Bool"("DisabledEnum"=w3638) -> ()  [unwired: 2 in, 2 out]
        n1913 = property on="Set from Input ch4" class="Bool"("DisabledEnum"=w3638) -> ()  [unwired: 2 in, 2 out]
      }
      event "Copy to Input ch2": Value Change {
        w3673 = T12."Enabled" ("Disabled")
        n1914 = event-data() -> ()  [unwired: 1 in, 6 out]
        n1915 = call "Read AcquisitionB.vi"("error in (no error)"=w3706, "S4ACS_GUI in"=w3707) -> ("error out"=w3702:errorcluster, "Acquisition.lvclass"=w3705:refnum<class "Acquisition.lvclass">, "S4ACS_GUI out"=w3674:refnum<class "S4GUI.lvclass">)  [unwired: 7 in]
        n1916 = call-dynamic "Read Channel.vi"("error in (no error)"=w3702, "Acquisition in"=w3705) -> ("error out"=w3701:errorcluster, "Channel.lvclass"=w3704:refnum<class "Channel.lvclass">)  [unwired: 7 in, 1 out]
        n1917 = call-dynamic "Read Interface.vi"("error in (no error)"=w3701, "Channel in"=w3704) -> ("error out"=w3700:errorcluster, "Interface.lvclass"=w3703:refnum<class "Interface.lvclass">)  [unwired: 7 in, 1 out]
        n1918 = call-dynamic "Get CCD_Config.vi"("error in (no error)"=w3700, "Interface in"=w3703) -> ("error out"=w3697:errorcluster, "output cluster"=w3696:T31)  [unwired: 7 in, 1 out]
        n1919 = Unbundle By Name(w3696) -> ("INITIAL_LINE"=w3695:u16, "INITIAL_COLUMN"=w3694:u16, "FINAL_LINE"=w3693:u16, "FINAL_COLUMN"=w3692:u16, "VBIN"=w3691:u16, "HBIN"=w3690:u16, "PREAMP"=w3689:u8, "EM_GAIN"=w3688:u16, "READOUT_RATE"=w3687:u8, "SHUTTER_OPENING_TIME"=w3686:u16, "SHUTTER_CLOSING_TIME"=w3685:u16, "VERTICAL_SHIFT_SPEED"=w3684:u8, "READ_MODE"=w3683:u8, "VERTICAL_CLOCK_VOLTAGE"=w3682:u8, "AD_CHANNEL"=w3681:u32, "SHUTTER_MODE"=w3680:u8, "SHUTTER_TTL"=w3679:u8, "TRIGGER_MODE"=w3678:u8, "FRAME_TRANSFER"=w3677:bool, "ACQUISITION_MODE"=w3676:u8, "EM_MODE"=w3675:u8)
        n1920 = local read "Input Cluster"() -> (w3699:T8)
        n1921 = Bundle By Name(cluster=w3699, "Parameters.Image \nInitial Line"=w3695, "Parameters.Image\nInitial Column"=w3694, "Parameters.Image\nFinal Line"=w3693, "Parameters.Image\nFInal Column"=w3692, "Parameters.Vertical\nBinning"=w3691, "Parameters.Horizontal\nBinning"=w3690, "Parameters.Pre-amplification\nGain"=w3689, "Parameters.CCD\nEM Gain"=w3688, "Parameters.Readout\nRate"=w3687, "Parameters.Shutter\nOpenning Time"=w3686, "Parameters.Shutter\nClosing Time"=w3685, "Parameters.Vertical\nShift Speed"=w3684, "Parameters.Read\nMode"=w3683, "Parameters.Vertical\nClock Voltage"=w3682, "Parameters.A/D \nChannel"=w3681, "Parameters.Shutter\nMode"=w3680, "Parameters.Shutter\nTTL"=w3679, "Parameters.Trigger\nMode"=w3678, "Parameters.Frame\nTransfer"=w3677, "Parameters.Acquisition\nMode"=w3676, "Parameters.CCD \nEM Mode"=w3675) -> (w3698:T8)
        n1922 = local write "Input Cluster"(w3698) -> ()
        n1923 = property on="Set from Input ch1" class="Bool"("DisabledEnum"=w3673) -> ()  [unwired: 2 in, 2 out]
        n1924 = property on="Set from Input ch3" class="Bool"("DisabledEnum"=w3673) -> ()  [unwired: 2 in, 2 out]
        n1925 = property on="Set from Input ch2" class="Bool"("DisabledEnum"=w3673) -> ()  [unwired: 2 in, 2 out]
        n1926 = property on="Set from Input ch4" class="Bool"("DisabledEnum"=w3673) -> ()  [unwired: 2 in, 2 out]
      }
      event "Copy to Input ch3": Value Change {
        w3708 = T12."Enabled" ("Disabled")
        n1927 = event-data() -> ()  [unwired: 1 in, 6 out]
        n1928 = call-dynamic "Read AcquisitionC.vi"("error in (no error)"=w3741, "S4ACS_GUI in"=w3742) -> ("error out"=w3737:errorcluster, "Acquisition.lvclass"=w3740:refnum<class "Acquisition.lvclass">, "S4ACS_GUI out"=w3709:refnum<class "S4GUI.lvclass">)  [unwired: 7 in]
        n1929 = call-dynamic "Read Channel.vi"("error in (no error)"=w3737, "Acquisition in"=w3740) -> ("error out"=w3736:errorcluster, "Channel.lvclass"=w3739:refnum<class "Channel.lvclass">)  [unwired: 7 in, 1 out]
        n1930 = call-dynamic "Read Interface.vi"("error in (no error)"=w3736, "Channel in"=w3739) -> ("error out"=w3735:errorcluster, "Interface.lvclass"=w3738:refnum<class "Interface.lvclass">)  [unwired: 7 in, 1 out]
        n1931 = call-dynamic "Get CCD_Config.vi"("error in (no error)"=w3735, "Interface in"=w3738) -> ("error out"=w3732:errorcluster, "output cluster"=w3731:T31)  [unwired: 7 in, 1 out]
        n1932 = Unbundle By Name(w3731) -> ("INITIAL_LINE"=w3730:u16, "INITIAL_COLUMN"=w3729:u16, "FINAL_LINE"=w3728:u16, "FINAL_COLUMN"=w3727:u16, "VBIN"=w3726:u16, "HBIN"=w3725:u16, "PREAMP"=w3724:u8, "EM_GAIN"=w3723:u16, "READOUT_RATE"=w3722:u8, "SHUTTER_OPENING_TIME"=w3721:u16, "SHUTTER_CLOSING_TIME"=w3720:u16, "VERTICAL_SHIFT_SPEED"=w3719:u8, "READ_MODE"=w3718:u8, "VERTICAL_CLOCK_VOLTAGE"=w3717:u8, "AD_CHANNEL"=w3716:u32, "SHUTTER_MODE"=w3715:u8, "SHUTTER_TTL"=w3714:u8, "TRIGGER_MODE"=w3713:u8, "FRAME_TRANSFER"=w3712:bool, "ACQUISITION_MODE"=w3711:u8, "EM_MODE"=w3710:u8)
        n1933 = local read "Input Cluster"() -> (w3734:T8)
        n1934 = Bundle By Name(cluster=w3734, "Parameters.Image \nInitial Line"=w3730, "Parameters.Image\nInitial Column"=w3729, "Parameters.Image\nFinal Line"=w3728, "Parameters.Image\nFInal Column"=w3727, "Parameters.Vertical\nBinning"=w3726, "Parameters.Horizontal\nBinning"=w3725, "Parameters.Pre-amplification\nGain"=w3724, "Parameters.CCD\nEM Gain"=w3723, "Parameters.Readout\nRate"=w3722, "Parameters.Shutter\nOpenning Time"=w3721, "Parameters.Shutter\nClosing Time"=w3720, "Parameters.Vertical\nShift Speed"=w3719, "Parameters.Read\nMode"=w3718, "Parameters.Vertical\nClock Voltage"=w3717, "Parameters.A/D \nChannel"=w3716, "Parameters.Shutter\nMode"=w3715, "Parameters.Shutter\nTTL"=w3714, "Parameters.Trigger\nMode"=w3713, "Parameters.Frame\nTransfer"=w3712, "Parameters.Acquisition\nMode"=w3711, "Parameters.CCD \nEM Mode"=w3710) -> (w3733:T8)
        n1935 = local write "Input Cluster"(w3733) -> ()
        n1936 = property on="Set from Input ch1" class="Bool"("DisabledEnum"=w3708) -> ()  [unwired: 2 in, 2 out]
        n1937 = property on="Set from Input ch3" class="Bool"("DisabledEnum"=w3708) -> ()  [unwired: 2 in, 2 out]
        n1938 = property on="Set from Input ch2" class="Bool"("DisabledEnum"=w3708) -> ()  [unwired: 2 in, 2 out]
        n1939 = property on="Set from Input ch4" class="Bool"("DisabledEnum"=w3708) -> ()  [unwired: 2 in, 2 out]
      }
      event "Copy to Input ch4": Value Change {
        w3743 = T12."Enabled" ("Disabled")
        n1940 = event-data() -> ()  [unwired: 1 in, 6 out]
        n1941 = call-dynamic "Read AcquisitionD.vi"("error in (no error)"=w3776, "S4ACS_GUI in"=w3777) -> ("error out"=w3772:errorcluster, "Acquisition.lvclass"=w3775:refnum<class "Acquisition.lvclass">, "S4ACS_GUI out"=w3744:refnum<class "S4GUI.lvclass">)  [unwired: 7 in]
        n1942 = call-dynamic "Read Channel.vi"("error in (no error)"=w3772, "Acquisition in"=w3775) -> ("error out"=w3771:errorcluster, "Channel.lvclass"=w3774:refnum<class "Channel.lvclass">)  [unwired: 7 in, 1 out]
        n1943 = call-dynamic "Read Interface.vi"("error in (no error)"=w3771, "Channel in"=w3774) -> ("error out"=w3770:errorcluster, "Interface.lvclass"=w3773:refnum<class "Interface.lvclass">)  [unwired: 7 in, 1 out]
        n1944 = call-dynamic "Get CCD_Config.vi"("error in (no error)"=w3770, "Interface in"=w3773) -> ("error out"=w3767:errorcluster, "output cluster"=w3766:T31)  [unwired: 7 in, 1 out]
        n1945 = Unbundle By Name(w3766) -> ("INITIAL_LINE"=w3765:u16, "INITIAL_COLUMN"=w3764:u16, "FINAL_LINE"=w3763:u16, "FINAL_COLUMN"=w3762:u16, "VBIN"=w3761:u16, "HBIN"=w3760:u16, "PREAMP"=w3759:u8, "EM_GAIN"=w3758:u16, "READOUT_RATE"=w3757:u8, "SHUTTER_OPENING_TIME"=w3756:u16, "SHUTTER_CLOSING_TIME"=w3755:u16, "VERTICAL_SHIFT_SPEED"=w3754:u8, "READ_MODE"=w3753:u8, "VERTICAL_CLOCK_VOLTAGE"=w3752:u8, "AD_CHANNEL"=w3751:u32, "SHUTTER_MODE"=w3750:u8, "SHUTTER_TTL"=w3749:u8, "TRIGGER_MODE"=w3748:u8, "FRAME_TRANSFER"=w3747:bool, "ACQUISITION_MODE"=w3746:u8, "EM_MODE"=w3745:u8)
        n1946 = local read "Input Cluster"() -> (w3769:T8)
        n1947 = Bundle By Name(cluster=w3769, "Parameters.Image \nInitial Line"=w3765, "Parameters.Image\nInitial Column"=w3764, "Parameters.Image\nFinal Line"=w3763, "Parameters.Image\nFInal Column"=w3762, "Parameters.Vertical\nBinning"=w3761, "Parameters.Horizontal\nBinning"=w3760, "Parameters.Pre-amplification\nGain"=w3759, "Parameters.CCD\nEM Gain"=w3758, "Parameters.Readout\nRate"=w3757, "Parameters.Shutter\nOpenning Time"=w3756, "Parameters.Shutter\nClosing Time"=w3755, "Parameters.Vertical\nShift Speed"=w3754, "Parameters.Read\nMode"=w3753, "Parameters.Vertical\nClock Voltage"=w3752, "Parameters.A/D \nChannel"=w3751, "Parameters.Shutter\nMode"=w3750, "Parameters.Shutter\nTTL"=w3749, "Parameters.Trigger\nMode"=w3748, "Parameters.Frame\nTransfer"=w3747, "Parameters.Acquisition\nMode"=w3746, "Parameters.CCD \nEM Mode"=w3745) -> (w3768:T8)
        n1948 = local write "Input Cluster"(w3768) -> ()
        n1949 = property on="Set from Input ch1" class="Bool"("DisabledEnum"=w3743) -> ()  [unwired: 2 in, 2 out]
        n1950 = property on="Set from Input ch3" class="Bool"("DisabledEnum"=w3743) -> ()  [unwired: 2 in, 2 out]
        n1951 = property on="Set from Input ch2" class="Bool"("DisabledEnum"=w3743) -> ()  [unwired: 2 in, 2 out]
        n1952 = property on="Set from Input ch4" class="Bool"("DisabledEnum"=w3743) -> ()  [unwired: 2 in, 2 out]
      }
      event "Scrollbar": Value Change {
        (unwired) 765.0 ("BarOffset")
        (unwired) 1000.0 ("BarOffset")
